vi "Columns.vi"() -> (2 "Columns":T1)   [LabVIEW 2020, in "tests.lvlib" / "Test1.lvclass"]
uses:
  Test1.lvclass
  Columns.ctl
  <vilib>/IlluminatedG/IG Conditum Base/Conditum/Columns/Integer/Integer.lvclass
  Test1.lvclass/Test1.ctl
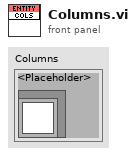
[diagram p1: front panel]
types:
  T1 = typedef "tests.lvlib/Test1.lvclass/Columns.ctl" = cluster{"<Placeholder>":refnum<class "Integer.lvclass">}
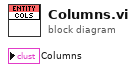
[diagram p0: block diagram]
diagram:
